vi "get_labview_versions.vi"(11 "error in (no error)":errorcluster) -> (4 "Version with path":T1[](array[typedef]), 6 "Versions":string[](array[string]), 15 "error out":errorcluster)   [LabVIEW 2023, in "task_6.lvlib"]
doc: "Get the versions and path of the labview installed."
uses:
  task_6.lvlib
  Controls/ver_path.ctl
  <vilib>/registry/registry.llb/Registry SAM.ctl
  <vilib>/registry/registry.llb/Read Registry Value Simple STR.vi
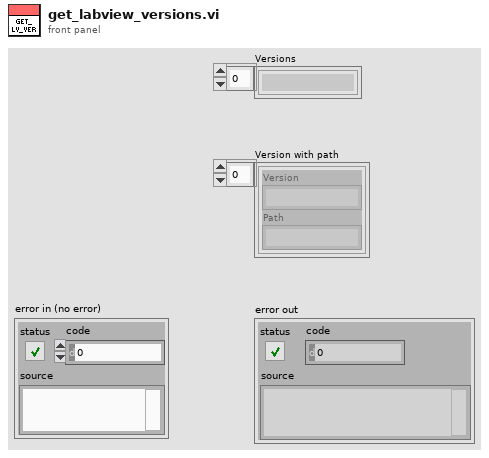
[diagram p1: front panel]
types:
  T1 = typedef "task_6.lvlib/ver_path.ctl" = cluster{"Version":string, "Path":string}
  T2 = cluster{"numSubKeys":i32, "maxSubKeyLen":i32, "maxSubKeyClassLen":i32}
  T3 = typedef "Registry SAM.ctl" = enum32{"KEY_QUERY_VALUE", "KEY_SET_VALUE", "KEY_CREATE_SUB_KEY", "KEY_ENUMERATE_SUB_KEYS", "KEY_NOTIFY", "KEY_CREATE_LINK", "KEY_READ", "KEY_WRITE", "KEY_ALL_ACCESS", "KEY_READ | KEY_WRITE"}
  T4 = typedef "Registry refnum.ctl" = refnum<k1>
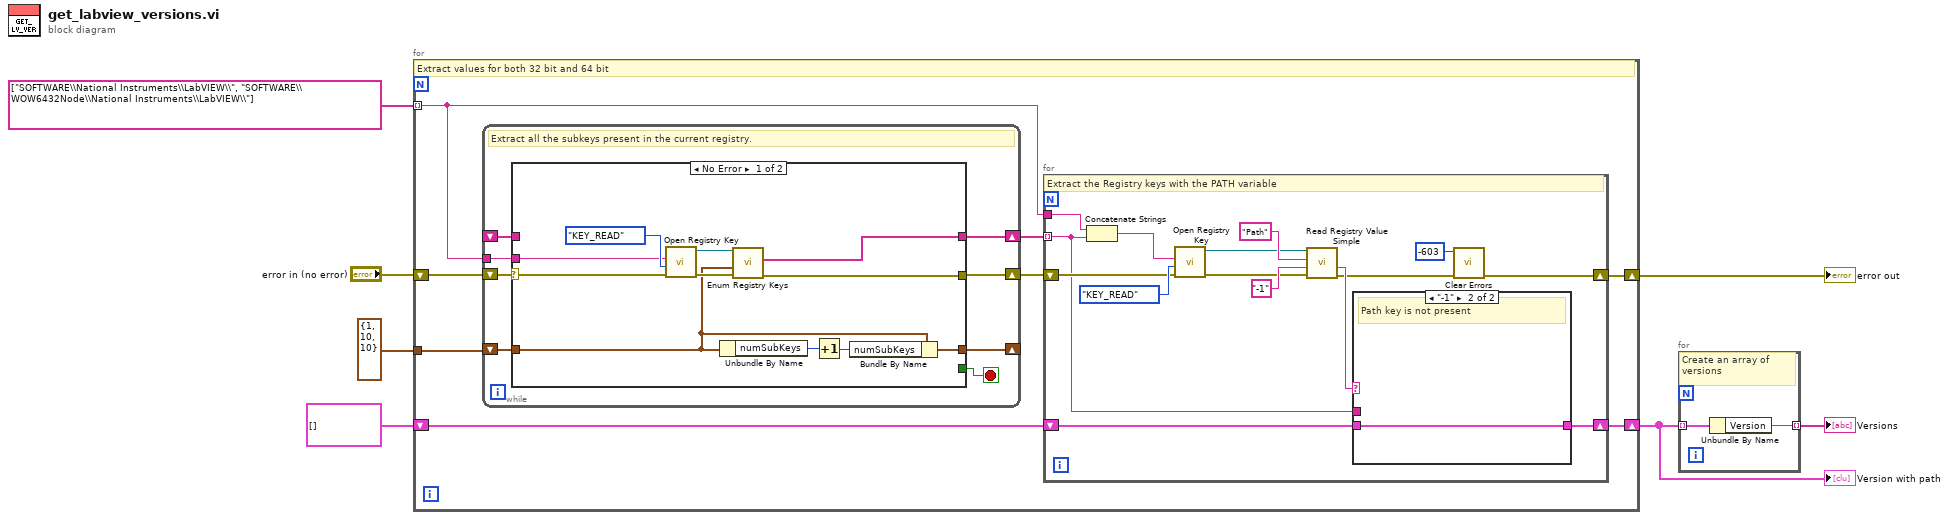
[diagram p0: block diagram]
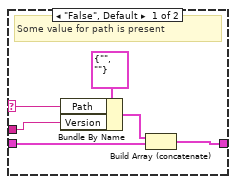
[diagram p2: hidden frame]
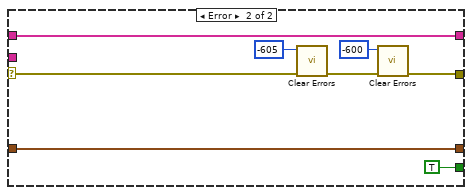
[diagram p3: hidden frame]
diagram:
  n1 = for {
    tunnel: T2 {"numSubKeys"=1, "maxSubKeyLen"=10, "maxSubKeyClassLen"=10} ("subkey info") -> [w14]
    tunnel: string[] ["SOFTWARE\\National Instruments\\LabVIEW\\", "SOFTWARE\\WOW6432Node\\National Instruments\\LabVIEW\\"] -> [w12] mode=indexing
    shift-right: [w10] -> w2
    shift-left: T1[] [] -> [w9]
    shift-right: [w8] -> w4
    shift-left: "error in (no error)" -> [w15]
    # "Extract values for both 32 bit and 64 bit"
    n2 = while {
      shift-right: [w42] -> _
      shift-left: w14 -> [w44]
      shift-right: [w41] -> w11
      shift-left: w15 -> [w45]
      tunnel: w12 -> [w43]
      shift-right: [w39] -> w13
      shift-left: _ -> [w38]
      stop <- w40 stop-if-true
      # "Extract all the subkeys present in the current registry."
      n3 = case shown="No Error" w45 {
        selector: w45 -> [w53 w64]
        tunnel: w44 -> [w50 w63]
        tunnel: w43 -> [w52 _]
        tunnel: [w49 w63] -> w42
        tunnel: [w47 w58] -> w41
        tunnel: [_ TRUE] -> w40
        tunnel: [w46 w59] -> w39
        tunnel: w38 -> [_ w59]
        frame No Error {
          n4 = call <vilib>:"Open Registry Key.vi"("error in (no error)"=w53, "security access mask (KEY_READ | KEY_WRITE)"=Registry_SAM."KEY_READ", "subkey"=w52) -> ("error out"=w55:errorcluster, "refnum out"=w56:T4)  [unwired: 7 in]
          n5 = Unbundle By Name(w50) -> ("numSubKeys"=w51:i32)
          n6 = call <vilib>:"Enum Registry Keys.vi"("error in (no error)"=w55, "subkey info"=w50, "refnum"=w56) -> ("error out"=w47:errorcluster, "subkeys"=w46:string[])  [unwired: 6 in, 1 out]
          n7 = Increment(x=w51) -> (x+1=w48:i32)
          n8 = Bundle By Name(cluster=w50, "numSubKeys"=w48) -> (w49:T2)
        }
        frame Error {
          n9 = call <vilib>:"Clear Errors.vi"("error in (no error)"=w64, "specific error code to clear (0: all)"=-605) -> ("error out"=w62:errorcluster)  [unwired: 4 in, 1 out]
          n10 = call <vilib>:"Clear Errors.vi"("error in (no error)"=w62, "specific error code to clear (0: all)"=-600) -> ("error out"=w58:errorcluster)  [unwired: 4 in, 1 out]
        }
      }
    }
    n11 = for {
      tunnel: w13 -> [w19] mode=indexing
      tunnel: w12 -> [w24]
      shift-right: [w21] -> w10
      shift-left: w9 -> [w20]
      shift-right: [w17] -> w8
      shift-left: w11 -> [w26]
      # "Extract the Registry keys with the PATH variable"
      n12 = Concatenate Strings(w24, w19) -> (w23:string)
      n13 = call <vilib>:"Open Registry Key.vi"("error in (no error)"=w26, "security access mask (KEY_READ | KEY_WRITE)"=Registry_SAM."KEY_READ", "subkey"=w23) -> ("error out"=w27:errorcluster, "refnum out"=w25:T4)  [unwired: 7 in]
      n14 = call-poly <vilib>:"Read Registry Value Simple.vi"("error in (no error)"=w27, "default data"="-1", "value"="Path", "refnum"=w25) -> ("error out"=w18:errorcluster, "String/Binary data"=w22:string)  [unwired: 2 in, 2 out]
      n15 = case shown="\"-1\"" w22 {
        selector: w22 -> [w35 _]
        tunnel: [w31 w37] -> w21
        tunnel: w20 -> [w32 w37]
        tunnel: w19 -> [w34 _]
        frame "False", Default {
          # "Some value for path is present"
          n16 = Bundle By Name(cluster=T1 {"Version"="", "Path"=""}, "Path"=w35, "Version"=w34) -> (w33:T1)
          n17 = Build Array (concatenate)(w33, w32) -> (w31:T1[])
        }
        frame "-1" {
          # "Path key is not present"
        }
      }
      n18 = call <vilib>:"Clear Errors.vi"("error in (no error)"=w18, "specific error code to clear (0: all)"=-603) -> ("error out"=w17:errorcluster)  [unwired: 4 in, 1 out]
    }
  }
  "error out" <- w4
  "Version with path" <- w2
  n19 = for {
    tunnel: w2 -> [w66] mode=indexing
    tunnel: [w65] -> w1 mode=indexing
    # "Create an array of versions"
    n20 = Unbundle By Name(w66) -> ("Version"=w65:string)
  }
  "Versions" <- w1
